vi "Get RTPath String Array.vi"(8 "error in (no error)":errorcluster, 11 "SysDef Log File Path":path) -> (0 "error out":errorcluster, 2 "File Path String Array":string[](array[string]))   [LabVIEW 2026, in "Telemetry System Tests.lvclass"]
uses:
  Telemetry System Tests.lvclass
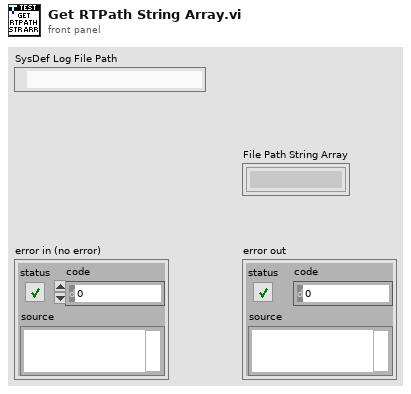
[diagram p1: front panel]
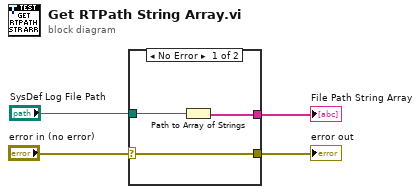
[diagram p0: block diagram]
diagram:
  n1 = case shown="No Error" "error in (no error)" {
    selector: "error in (no error)" -> [w7 w8]
    tunnel: [w7 w8] -> w4
    tunnel: [w5 _] -> w3
    tunnel: "SysDef Log File Path" -> [w6 _]
    frame No Error {
      n2 = Path to Array of Strings(0:w6) -> (2:w5:string[])  [unwired: 1 out]
    }
    frame Error {
    }
  }
  "error out" <- w4
  "File Path String Array" <- w3
